vi "Read Trace Statistics.vi"(8 "error in (no error)":errorcluster, 10 "Channel (1)":i32=1, 11 "VISA resource name":refnum<visa-resource-name>) -> (0 "error out":errorcluster, 2 "Data":dbl, 3 "VISA resource name out":refnum<visa-resource-name>)   [LabVIEW 2018, in "Keysight PNA Series.lvlib"]
doc: "Reads the trace statistic data for the selected statistic type for the specified channel."
uses:
  Keysight PNA Series.lvlib
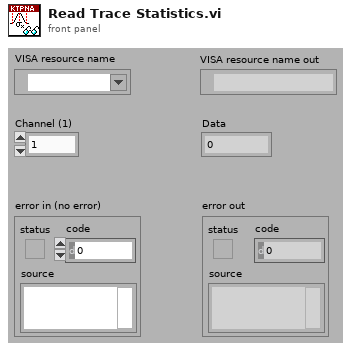
[diagram p1: front panel]
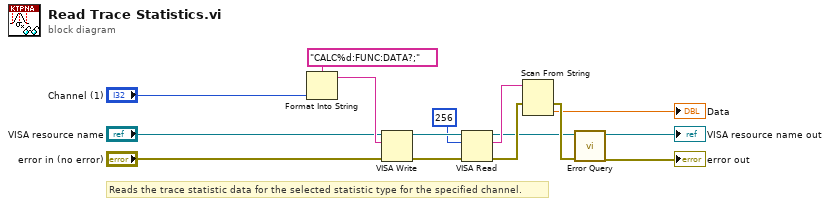
[diagram p0: block diagram]
diagram:
  # "Reads the trace statistic data for the selected statistic type for the specified channel."
  n1 = Format Into String(format string="CALC%d:FUNC:DATA?;", "Channel (1)") -> (resulting string=w13:string)  [unwired: 2 in, 1 out]
  n2 = VISA Write(VISA resource name="VISA resource name", write buffer=w13, error in (no error)="error in (no error)") -> (VISA resource name out=w7:refnum<visa-resource-name>, error out=w8:errorcluster)  [unwired: 1 out]
  n3 = VISA Read(VISA resource name=w7, byte count=u32 256, error in (no error)=w8) -> (VISA resource name out=w1:refnum<visa-resource-name>, read buffer=w2:string, error out=w5:errorcluster)  [unwired: 1 out]
  n4 = Scan From String(input string=w2, error in=w5) -> (error out=w4:errorcluster, output 1=→"Data":dbl)  [unwired: 3 in, 2 out]
  n5 = call "Error Query.vi"("error in (no error)"=w4, "VISA resource name"=w1) -> ("error out"=→"error out":errorcluster, "VISA resource name out"=→"VISA resource name out":refnum<visa-resource-name>)  [unwired: 6 in, 2 out]
